vi "Task - Pressure & Flow.vi"() -> ()   [LabVIEW 2013]
panel:
  in  "stop":bool
  out "MKS946 High Pressure\n(Torr)":dbl
  out "Target Cavity Flow\n(SCCM)":dbl
  out "Separator Flow\n(SCCM)":dbl
  out "Baratron\n(Torr)":dbl
  in  "MKS 670 VISA In":refnum<visa-resource-name>
  in  "MKS 946 VISA In":refnum<visa-resource-name>
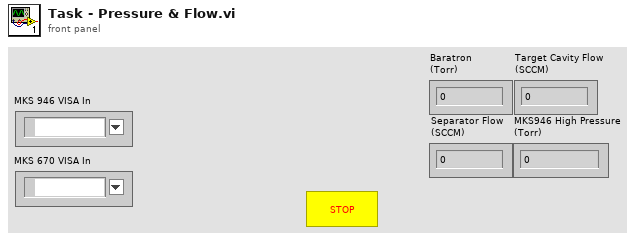
[diagram p1: front panel]
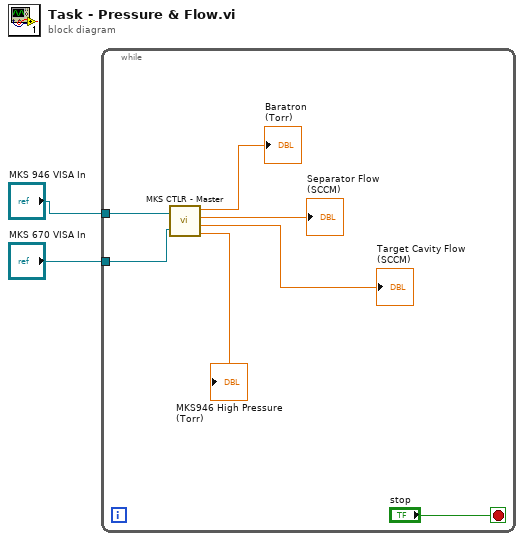
[diagram p0: block diagram]
diagram:
  n1 = while {
    tunnel: "MKS 946 VISA In" -> [w9]
    tunnel: "MKS 670 VISA In" -> [w8]
    stop <- "stop" stop-if-true
    n2 = call "MKS CTLR - Master.vi"("MKS 946 VISA In"=w9, "MKS 670 VISA In"=w8) -> ("Baratron\n(Torr)"=→"Baratron\n(Torr)":dbl, "Separator Flow\n(SCCM)"=→"Separator Flow\n(SCCM)":dbl, "Target Cavity Flow\n(SCCM)"=→"Target Cavity Flow\n(SCCM)":dbl, "MKS946 High Pressure\n(Torr)"=→"MKS946 High Pressure\n(Torr)":dbl)
  }
